vi "Configure Serial Bus (LIN - Trigger).vi"(0 "VISA resource name":refnum<visa-resource-name>, 1 "Data Pattern (0)":string="0", 2 "Data Length (4 Bytes)":dbl=4.0, 5 "Serial Bus Name (1: Serial Bus 1)":i32(ring)=1 items=["Serial Bus 1"=1, "Serial Bus 2"=2], 7 "Trigger Condition (0: Sync Break)":i32(ring) items=["Sync Break", "ID", "Data", "Frame", "Frame and Signal"], 9 "Frame ID (-1)":i32=-1, 11 "error in (no error)":errorcluster, 12 "Data Pattern Base (0: Binary)":i32(ring) items=["Binary", "Hex", "Decimal"]) -> (4 "VISA resource name out":refnum<visa-resource-name>, 15 "error out":errorcluster)   [LabVIEW 2016, in "Agilent 2000 3000 X-Series.lvlib"]
doc: "Configures the trigger settings of LIN bus."
uses:
  Agilent 2000 3000 X-Series.lvlib
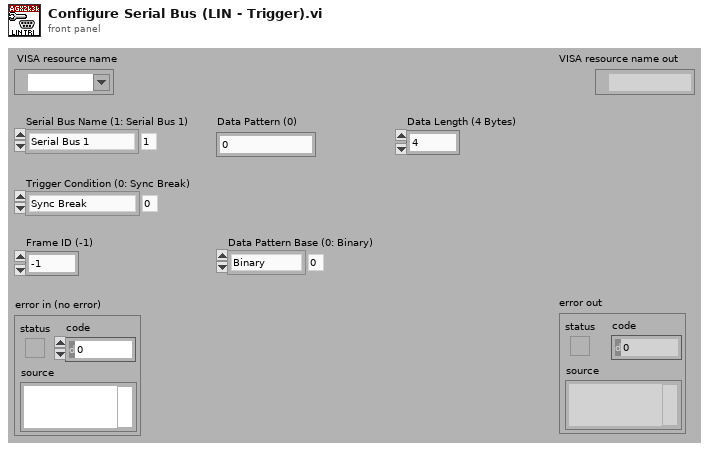
[diagram p1: front panel]
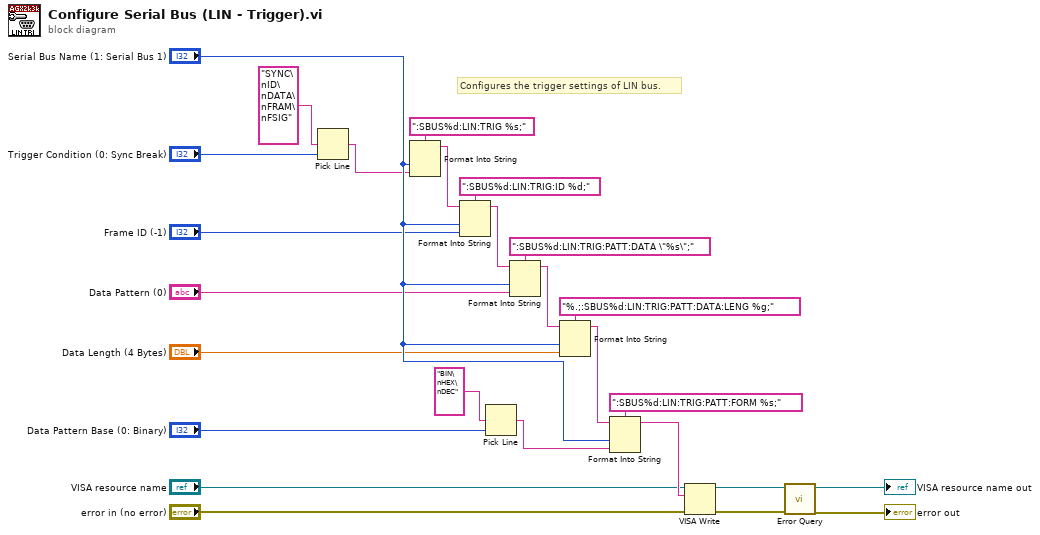
[diagram p0: block diagram]
diagram:
  # "Configures the trigger settings of LIN bus."
  n1 = Pick Line(multi-line string="SYNC\nID\nDATA\nFRAM\nFSIG", line index="Trigger Condition (0: Sync Break)") -> (output string=w22:string)  [unwired: 1 out]
  n2 = Format Into String(format string=":SBUS%d:LIN:TRIG %s;", "Serial Bus Name (1: Serial Bus 1)", w22) -> (resulting string=w21:string)  [unwired: 2 in, 1 out]
  n3 = Format Into String(format string=":SBUS%d:LIN:TRIG:ID %d;", initial string=w21, "Serial Bus Name (1: Serial Bus 1)", "Frame ID (-1)") -> (resulting string=w18:string)  [unwired: 1 in, 1 out]
  n4 = Pick Line(multi-line string="BIN\nHEX\nDEC", line index="Data Pattern Base (0: Binary)") -> (output string=w8:string)  [unwired: 1 out]
  n5 = Format Into String(format string=":SBUS%d:LIN:TRIG:PATT:DATA \"%s\";", initial string=w18, "Serial Bus Name (1: Serial Bus 1)", "Data Pattern (0)") -> (resulting string=w15:string)  [unwired: 1 in, 1 out]
  n6 = Format Into String(format string="%.;:SBUS%d:LIN:TRIG:PATT:DATA:LENG %g;", initial string=w15, "Serial Bus Name (1: Serial Bus 1)", "Data Length (4 Bytes)") -> (resulting string=w10:string)  [unwired: 1 in, 1 out]
  n7 = Format Into String(format string=":SBUS%d:LIN:TRIG:PATT:FORM %s;", initial string=w10, "Serial Bus Name (1: Serial Bus 1)", w8) -> (resulting string=w7:string)  [unwired: 1 in, 1 out]
  n8 = VISA Write(VISA resource name="VISA resource name", write buffer=w7, error in (no error)="error in (no error)") -> (VISA resource name out=w4:refnum<visa-resource-name>, error out=w3:errorcluster)  [unwired: 1 out]
  n9 = call "Error Query.vi"("error in (no error)"=w3, "VISA resource name"=w4) -> ("error out"=→"error out":errorcluster, "VISA resource name out"=→"VISA resource name out":refnum<visa-resource-name>)  [unwired: 8 out]
